vi "Struct Add Element.vi"(9 "Element name":string="var1", 10 "Element type":string="double", 11 "String in":string) -> (3 "String out":string)   [LabVIEW 2014, in "C Header Generator.lvlib"]
uses:
  C Header Generator.lvlib
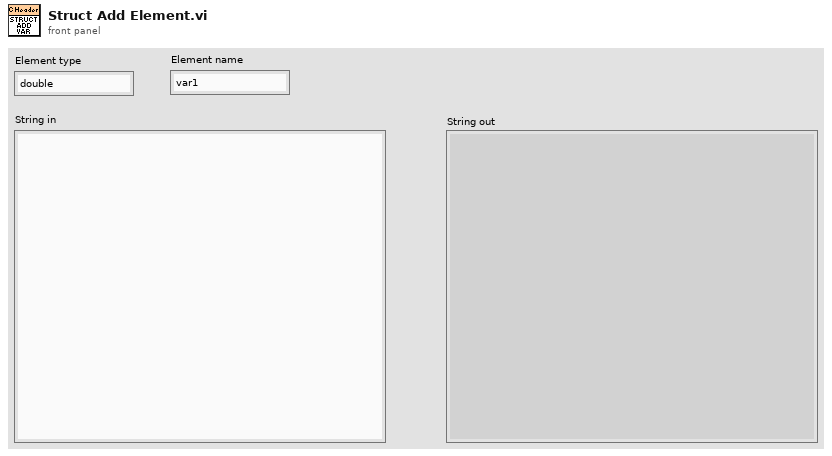
[diagram p1: front panel]
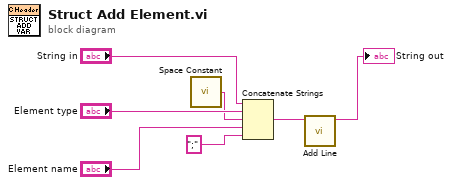
[diagram p0: block diagram]
diagram:
  n1 = call <vilib>:"Space Constant.vi"() -> ("String"=w6:string)
  n2 = Concatenate Strings("String in", "Element type", w6, "Element name", ";" ("string")) -> (w2:string)
  n3 = call "Add Line.vi"("String in"=w2) -> ("String out"=→"String out":string)  [unwired: 10 in]
